vi "叶绿素a校准.vi"() -> ()   [LabVIEW 2016, in "国弘多参数.lvlib"]
panel:
  out "测试值":dbl
  out "电极斜率":dbl
  out "电极零点":dbl
  # "叶绿素a电极设定"
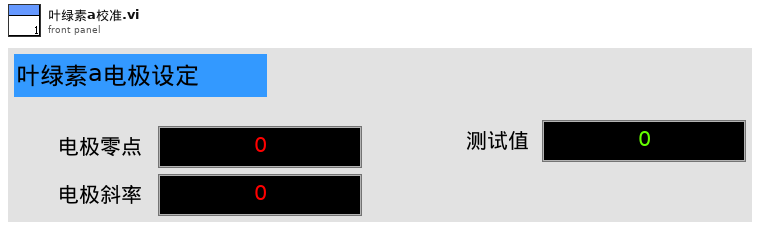
[diagram p1: front panel]
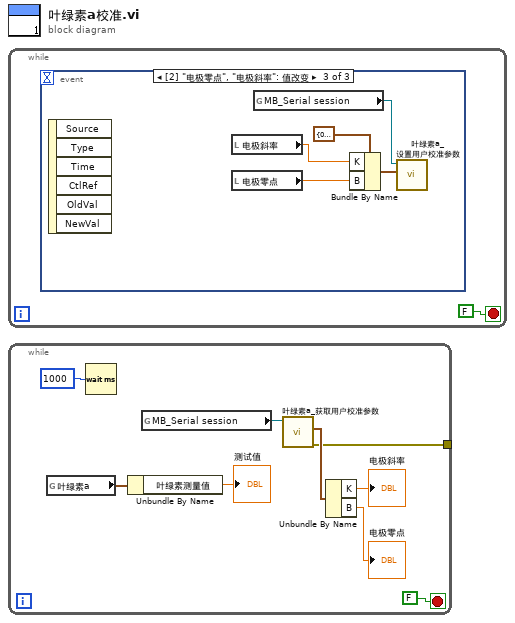
[diagram p0: block diagram]
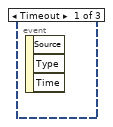
[diagram p2: hidden frame]
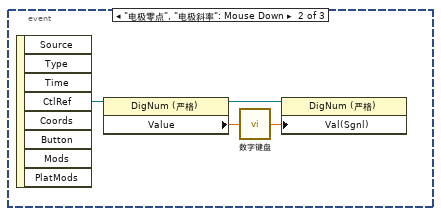
[diagram p3: hidden frame]
diagram:
  n1 = while {
    stop <- FALSE stop-if-true
    n2 = event shown="[2] \"电极零点\", \"电极斜率\": 值改变" {
      selector: _ -> [_ _ _]
      dyn-events: _ -> [_ _ _]
      timeout: _ -> [_ _ _]
      event Timeout {
        n3 = event-data() -> ()  [unwired: 1 in, 3 out]
      }
      event "电极零点", "电极斜率": Mouse Down {
        n4 = event-data() -> ("CtlRef"=w2:refnum<vi>)  [unwired: 1 in, 7 out]
        n5 = property class="DigNum (严格)"(reference=w2) -> (reference out=w3:refnum<vi>, "Value"=w4:dbl)  [unwired: 1 in, 1 out]
        n6 = call "数字键盘.vi"("OldNumber"=w4) -> ("NewNumber"=w5:sgl)
        n7 = property class="DigNum (严格)"(reference=w3, "Val(Sgnl)"=w5) -> ()  [unwired: 1 in, 2 out]
      }
      event "电极零点", "电极斜率": Value Change {
        n8 = event-data() -> ()  [unwired: 1 in, 6 out]
        n9 = local read "电极斜率"() -> (w7:dbl)
        n10 = local read "电极零点"() -> (w6:dbl)
        n11 = global read "过程全局变量.vi" "MB_Serial session"() -> (w10:refnum<class "MB_Master_Serial.lvclass">)
        n12 = Bundle By Name(cluster=cluster{"K":sgl, "B":sgl} {"K"=0.0, "B"=0.0} ("用户校准参数"), "K"=w7, "B"=w6) -> (w8:cluster{"K":sgl, "B":sgl})
        n13 = call "叶绿素a_设置用户校准参数.vi"("用户校准参数"=w8, "MB_Serial session in"=w10) -> ()  [unwired: 8 in, 2 out]
      }
    }
  }
  n14 = while {
    tunnel: [w13] -> _
    stop <- FALSE stop-if-true
    n15 = global read "过程全局变量.vi" "叶绿素a"() -> (w12:cluster{"温度测量值":sgl, "叶绿素测量值":sgl, "错误标志":u16})
    n16 = Wait (ms)(milliseconds to wait=u32 1000 ("等待时间（毫秒）")) -> ()  [unwired: 1 out]
    n17 = Unbundle By Name(w12) -> ("叶绿素测量值"=→"测试值":sgl)
    n18 = global read "过程全局变量.vi" "MB_Serial session"() -> (w17:refnum<class "MB_Master_Serial.lvclass">)
    n19 = call "叶绿素a_获取用户校准参数.vi"("MB_Serial session in"=w17) -> ("error out"=w13:errorcluster, "输出值"=w16:cluster{"K":sgl, "B":sgl})  [unwired: 8 in, 1 out]
    n20 = Unbundle By Name(w16) -> ("K"=→"电极斜率":sgl, "B"=→"电极零点":sgl)
  }
